vi "Read Export Data Locations.vi"(8 "error in (no error)":errorcluster, 11 "Harmonics_Relative_Power in":refnum<class "RxBN dBmHz Calculation.lvclass">=refnum) -> (0 "error out":errorcluster, 2 "Export Data Locations":string[](array[string]), 3 "Harmonics_Relative_Power out":refnum<class "RxBN dBmHz Calculation.lvclass">)   [LabVIEW 2016, in "SeqAuto Evaluations.lvlib" / "RxBN dBmHz Calculation.lvclass"]
uses:
  RxBN dBmHz Calculation.lvclass
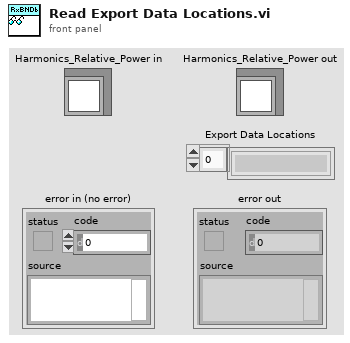
[diagram p1: front panel]
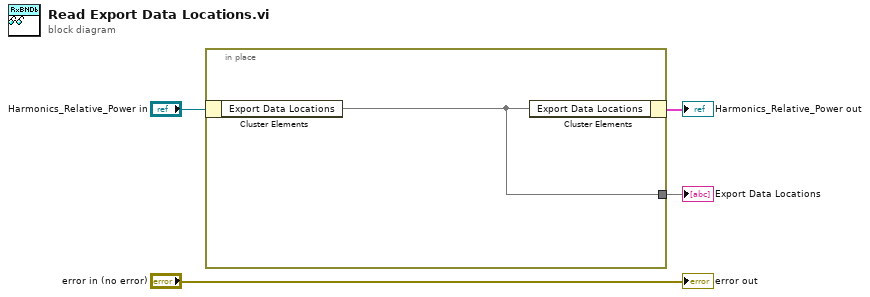
[diagram p0: block diagram]
diagram:
  n1 = in-place {
    in-place-border: [w5] -> w2
    n2 = in-place-cluster #1("Harmonics_Relative_Power in") -> ("Export Data Locations"=w5)
    n3 = in-place-cluster #1("Export Data Locations"=w5) -> (→"Harmonics_Relative_Power out":cluster{})
  }
  "Export Data Locations" <- w2
  "error out" <- "error in (no error)"
